vi "save_T2.vi"(3 "position_xyzt":T2, 5 "triggers":u32[][](array[numeric]), 6 "image_info":T1={"file_path"=path "", "file_name"="", "image"=[], "image_size_xy"={"image_size_x_um"=1.0, "image_size_y_um"=1.0}, "pixel_dwell_time_ms"=1.0, "Laser_power_mW"=1.0, "pixel_size"=0.0, "tile_ij"={"tile_i"=0, "tile_j"=0}, "Objective"="", "ColorMarkers"=[], "timestamp"=timestamp(0 s since 1904-01-01), "micro-position-xyz"={"micro-position_x_mm"=1.0, "micro-position_y_mm"=1.0, "micro-position_z_mm"=1.0}, "zero_xyz"={"zero_x_mm"=0.0, "zero_y_mm"=0.0, "zero_z_mm"=0.0}, "nano-position-xyz"={"nano-position_x_V"=1.0, "nano-position_y_V"=1.0, "nano-position_z_V"=1.0}, "Kxyz"={"Kx_V/um"=1.0, "Ky_V/um"=1.0, "Kz_V/um"=1.0}}, 7 "timetags":u32[][](array[numeric]), 8 "fitted_signal_in":T4 caption="fitted_signal", 9 "fit_parameters":T6 {"T1 2" format="%.3g"; "T1" format="%.3g"; "C1" format="%.3g"; "Tm" format="%.3g"; "Cm" format="%.3g"; "Ie" format="%.3g"}, 10 "T1_parameters":T3, 11 "T1_curve_in":T5) -> ()   [LabVIEW 2018]
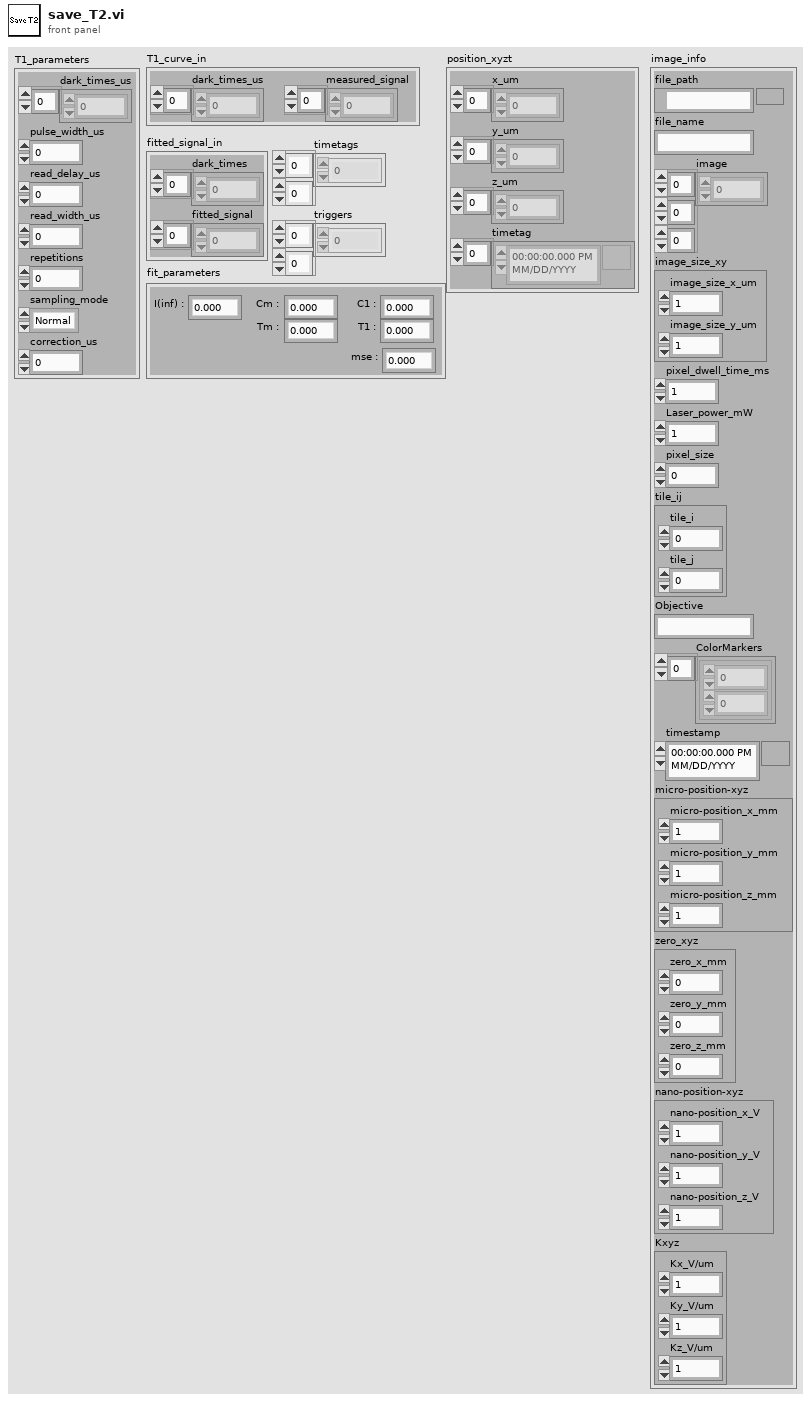
[diagram p1: front panel]
types:
  T1 = cluster{"file_path":path, "file_name":string, "image":dbl[][][], "image_size_xy":cluster{"image_size_x_um":sgl, "image_size_y_um":sgl}, "pixel_dwell_time_ms":sgl, "Laser_power_mW":sgl, "pixel_size":dbl, "tile_ij":cluster{"tile_i":i32, "tile_j":i32}, "Objective":string, "ColorMarkers":cluster{dbl, u32}[], "timestamp":timestamp, "micro-position-xyz":cluster{"micro-position_x_mm":sgl, "micro-position_y_mm":sgl, "micro-position_z_mm":sgl}, "zero_xyz":cluster{"zero_x_mm":dbl, "zero_y_mm":dbl, "zero_z_mm":dbl}, "nano-position-xyz":cluster{"nano-position_x_V":sgl, "nano-position_y_V":sgl, "nano-position_z_V":sgl}, "Kxyz":cluster{"Kx_V/um":sgl, "Ky_V/um":sgl, "Kz_V/um":sgl}}
  T2 = cluster{"x_um":sgl[], "y_um":sgl[], "z_um":sgl[], "timetag":timestamp[]}
  T3 = cluster{"dark_times_us":dbl[], "pulse_width_us":dbl, "read_delay_us":dbl, "read_width_us":dbl, "repetitions":i32, "sampling_mode":enum16{"Normal", "Sweep"}, "correction_us":dbl}
  T4 = cluster{"dark_times":dbl[], "fitted_signal":dbl[]}
  T5 = cluster{"dark_times_us":dbl[], "measured_signal":dbl[]}
  T6 = cluster{"Ie":dbl, "Cm":dbl, "Tm":dbl, "C1":dbl, "T1":dbl, "T1 2":dbl}
  T7 = enum16{"open", "replace", "create", "open or create", "replace or create", "replace or create with confirmation"}
  T8 = cluster{"x_um":sgl[], "y_um":sgl[], "z_um":sgl[], u32[]}
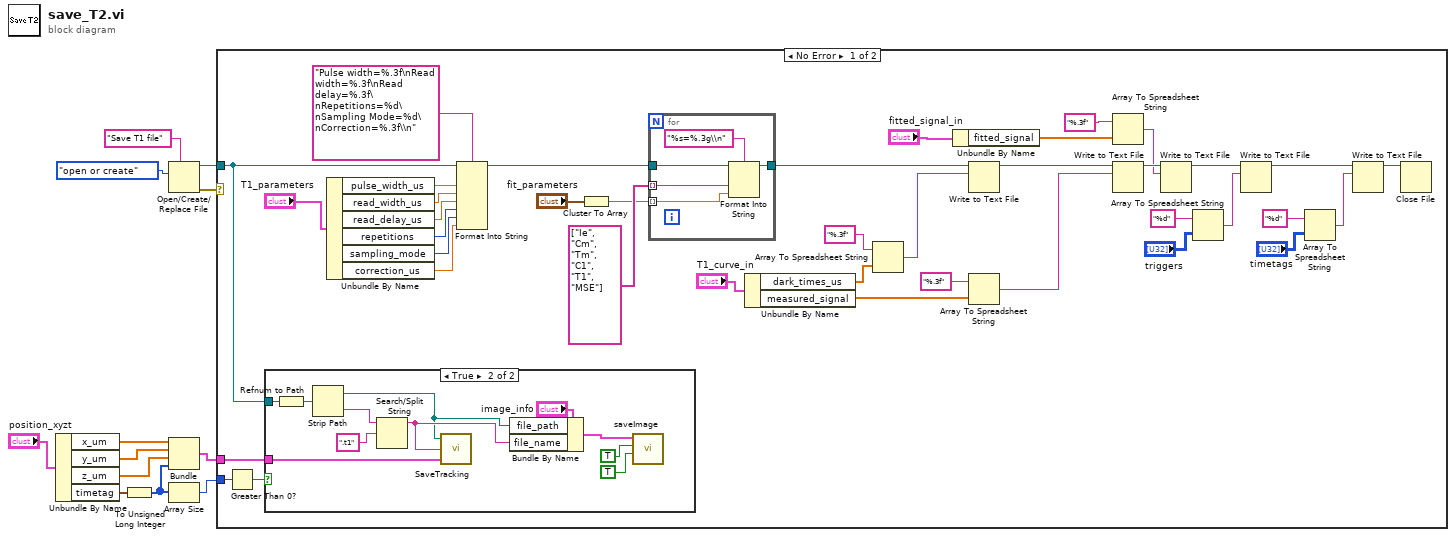
[diagram p0: block diagram]
diagram:
  n1 = Unbundle By Name("position_xyzt") -> ("x_um"=w6:sgl[], "y_um"=w7:sgl[], "z_um"=w8:sgl[], "timetag"=w5:timestamp[])
  n2 = To Unsigned Long Integer(number=w5) -> (unsigned 32bit integer=w2:u32[])
  n3 = Open/Create/Replace File(prompt="Save T1 file", operation (0:open)=T7."open or create") -> (refnum out=w11:refnum<file>, error out=w9:errorcluster)  [unwired: 4 in, 1 out]
  n4 = Bundle("x_um"=w6, "y_um"=w7, "z_um"=w8, w2) -> (w3:T8)  [unwired: 1 in]
  n5 = Array Size(array=w2) -> (size(s)=w1:i32)
  n6 = case shown="No Error" w9 {
    tunnel: w11 -> [w15 _]
    tunnel: w3 -> [w14 _]
    tunnel: w1 -> [w13 _]
    frame No Error {
      n7 = Greater Than 0?(x=w13) -> (x > 0?=w17:bool)
      n8 = case shown="True" w17 {
        tunnel: w14 -> [_ w62]
        tunnel: w15 -> [_ w60]
        frame False {
        }
        frame True {
          n9 = Refnum to Path(1:w60) -> (0:w61:path)
          n10 = Strip Path(path=w61) -> (stripped path=w56:path, name=w59:string)
          n11 = Search/Split String(string=w59, search string/char (-)=".t1") -> (substring before match=w57:string)  [unwired: 1 in, 2 out]
          n12 = call "SaveTracking.vi"("Input Data xyzt"=w62, "file_name"=w57, "file path (dialog if empty)"=w56) -> ()  [unwired: 1 in]
          n13 = Bundle By Name(cluster="image_info", "file_path"=w56, "file_name"=w57) -> (w55:T1)
          n14 = call "saveImage.vi"("save_txt"=TRUE, "save_tiff"=TRUE, "image_info"=w55) -> ()  [unwired: 9 in]
        }
      }
      n15 = Unbundle By Name("T1_parameters") -> ("pulse_width_us"=w37:dbl, "read_width_us"=w36:dbl, "read_delay_us"=w35:dbl, "repetitions"=w34:i32, "sampling_mode"=w24:enum16{"Normal", "Sweep"}, "correction_us"=w23:dbl)
      n16 = Format Into String(format string="Pulse width=%.3f\nRead width=%.3f\nRead delay=%.3f\nRepetitions=%d\nSampling Mode=%d\nCorrection=%.3f\\n", initial string=w15, w37, w36, w35, w34, w24, w23) -> (resulting string=w16:refnum<file>)  [unwired: 1 in, 1 out]
      n17 = Cluster To Array(cluster="fit_parameters") -> (array=w49:dbl[])
      n18 = for {
        tunnel: string[] ["Ie", "Cm", "Tm", "C1", "T1", "MSE"] -> [w66] mode=indexing
        tunnel: w49 -> [w65] mode=indexing
        tunnel: [w64] -> w33
        tunnel: w16 -> [w63]
        n19 = Format Into String(format string="%s=%.3g\\n", initial string=w63, w66, w65) -> (resulting string=w64:refnum<file>)  [unwired: 1 in, 1 out]
      }
      n20 = Unbundle By Name("T1_curve_in") -> ("dark_times_us"=w47:dbl[], "measured_signal"=w43:dbl[])
      n21 = Array To Spreadsheet String(array=w47, 3:"%.3f" ("format string")) -> (spreadsheet string=w30:string)  [unwired: 1 in]
      n22 = Unbundle By Name("fitted_signal_in") -> ("fitted_signal"=w42:dbl[])
      n23 = Write to Text File(file (use dialog)=w33, text=w30) -> (refnum out=w45:refnum<file>)  [unwired: 2 in, 2 out]
      n24 = Array To Spreadsheet String(array=w43, 3:"%.3f" ("format string")) -> (spreadsheet string=w32:string)  [unwired: 1 in]
      n25 = Array To Spreadsheet String(array=w42, 3:"%.3f" ("format string")) -> (spreadsheet string=w31:string)  [unwired: 1 in]
      n26 = Write to Text File(file (use dialog)=w45, text=w32) -> (refnum out=w40:refnum<file>)  [unwired: 2 in, 2 out]
      n27 = Write to Text File(file (use dialog)=w40, text=w31) -> (refnum out=w21:refnum<file>)  [unwired: 2 in, 2 out]
      n28 = Array To Spreadsheet String(array="triggers", 3:"%d" ("format string")) -> (spreadsheet string=w19:string)  [unwired: 1 in]
      n29 = Write to Text File(file (use dialog)=w21, text=w19) -> (refnum out=w20:refnum<file>)  [unwired: 2 in, 2 out]
      n30 = Array To Spreadsheet String(array="timetags", 3:"%d" ("format string")) -> (spreadsheet string=w28:string)  [unwired: 1 in]
      n31 = Write to Text File(file (use dialog)=w20, text=w28) -> (refnum out=w29:refnum<file>)  [unwired: 2 in, 2 out]
      n32 = Close File(refnum=w29) -> ()  [unwired: 1 in, 2 out]
    }
    frame Error {
    }
  }
